vi "QcpTest.vi"() -> ()   [LabVIEW 2017]
uses:
  <userlib>/836-Library/System/QCP_V2/QCPSupportCode/QcpTests.ctl
  <userlib>/836-Library/System/QCP_V2/QCPSupportCode/QCP_GetDbl.vi
  <userlib>/836-Library/System/QCP_V2/QCPSupportCode/QCP_GetDblArr.vi
  <userlib>/836-Library/System/QCP_V2/QCPSupportCode/QCP_SetDbl.vi
panel:
  out "Numeric":i32
  out "All Tests Passed":bool
  out "Last Test Run":T1
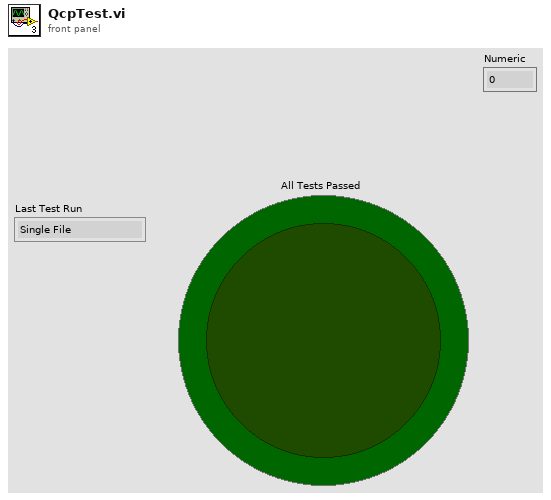
[diagram p1: front panel]
types:
  T1 = typedef "QcpTests.ctl" = enum16{"Single File", "Multiple FIle", "Tuning Mode", "Write FIle", "Same Name Prot On", "Same Name Prot Off", "NUM_TESTS"}
  T2 = typedef "QCP_RefNum.ctl" = cluster{"Data Value Refnum":refnum<data-value>, "semaphore":T3}
  T3 = typedef "Semaphore RefNum" = refnum<k1>
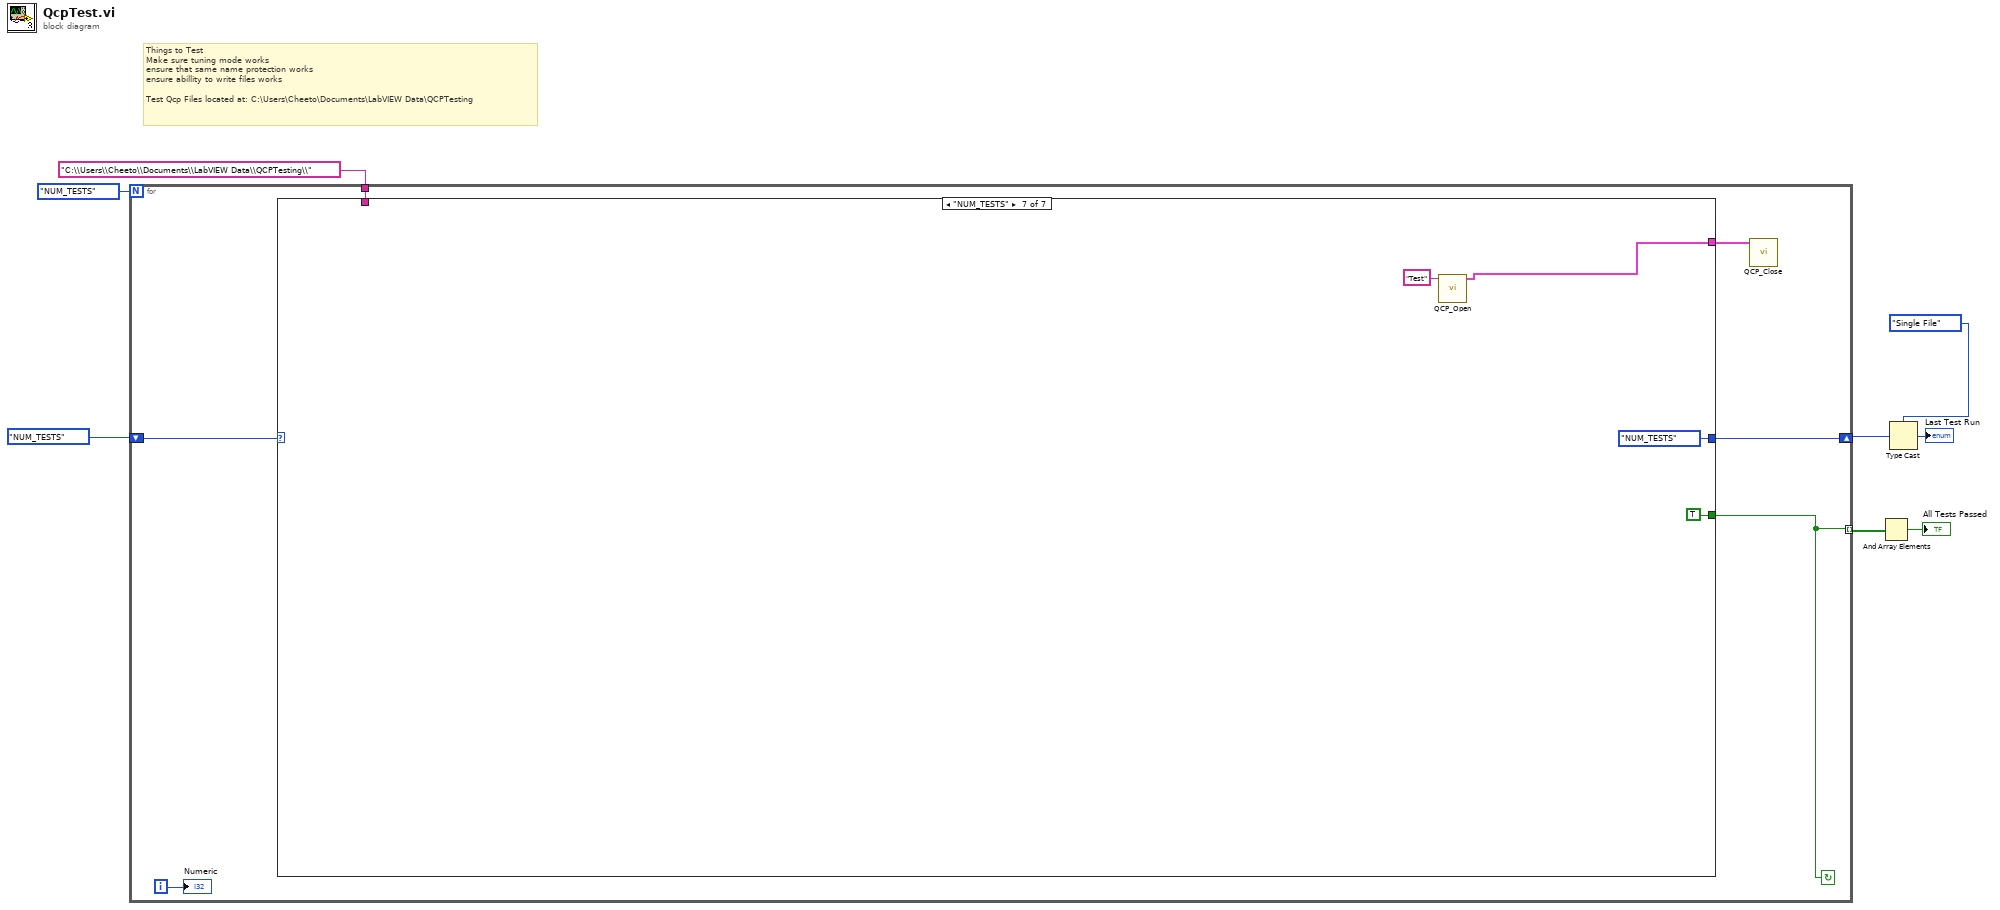
[diagram p0: block diagram]
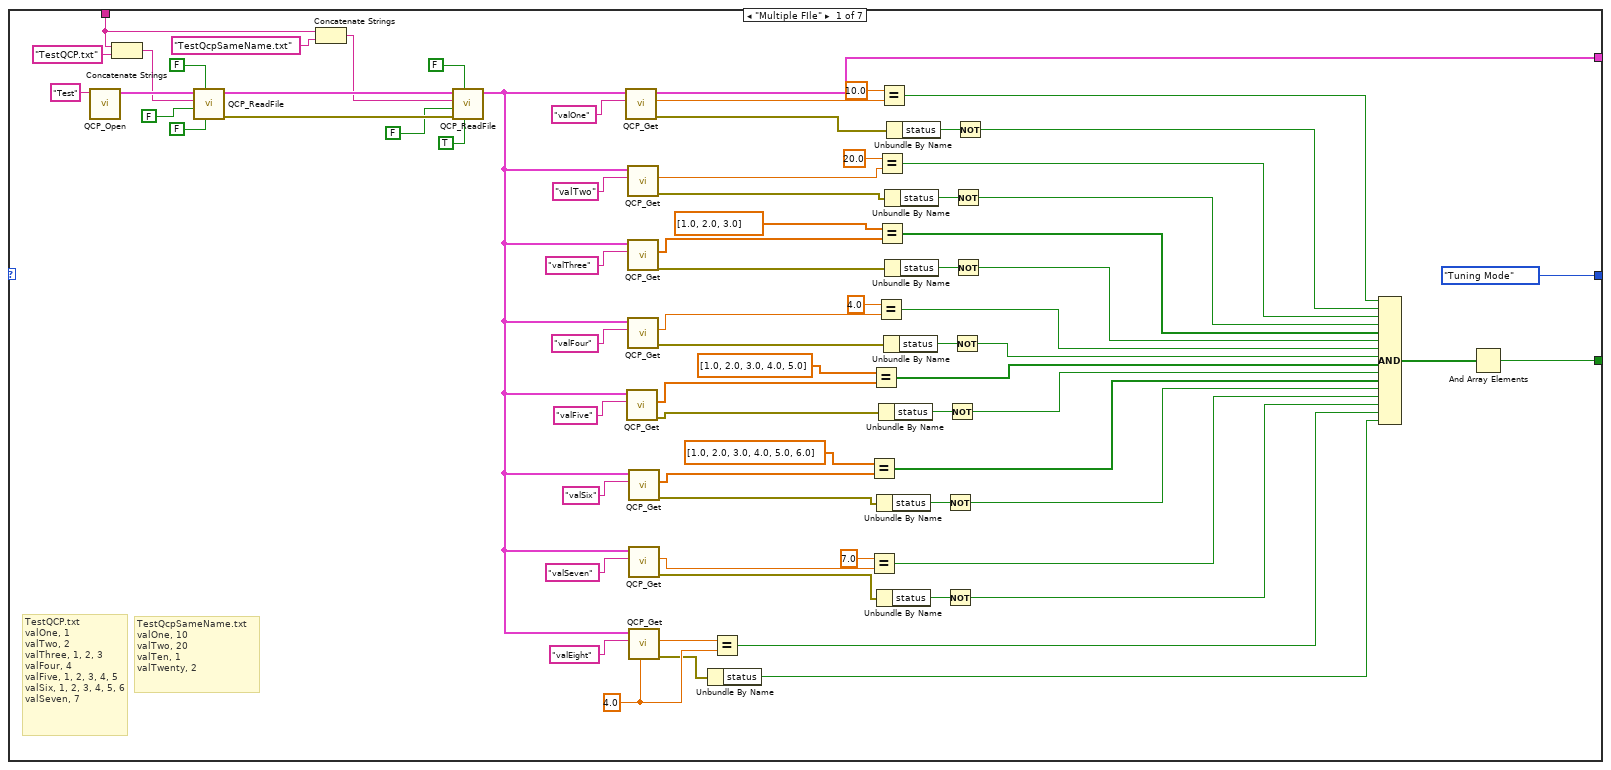
[diagram p2: hidden frame]
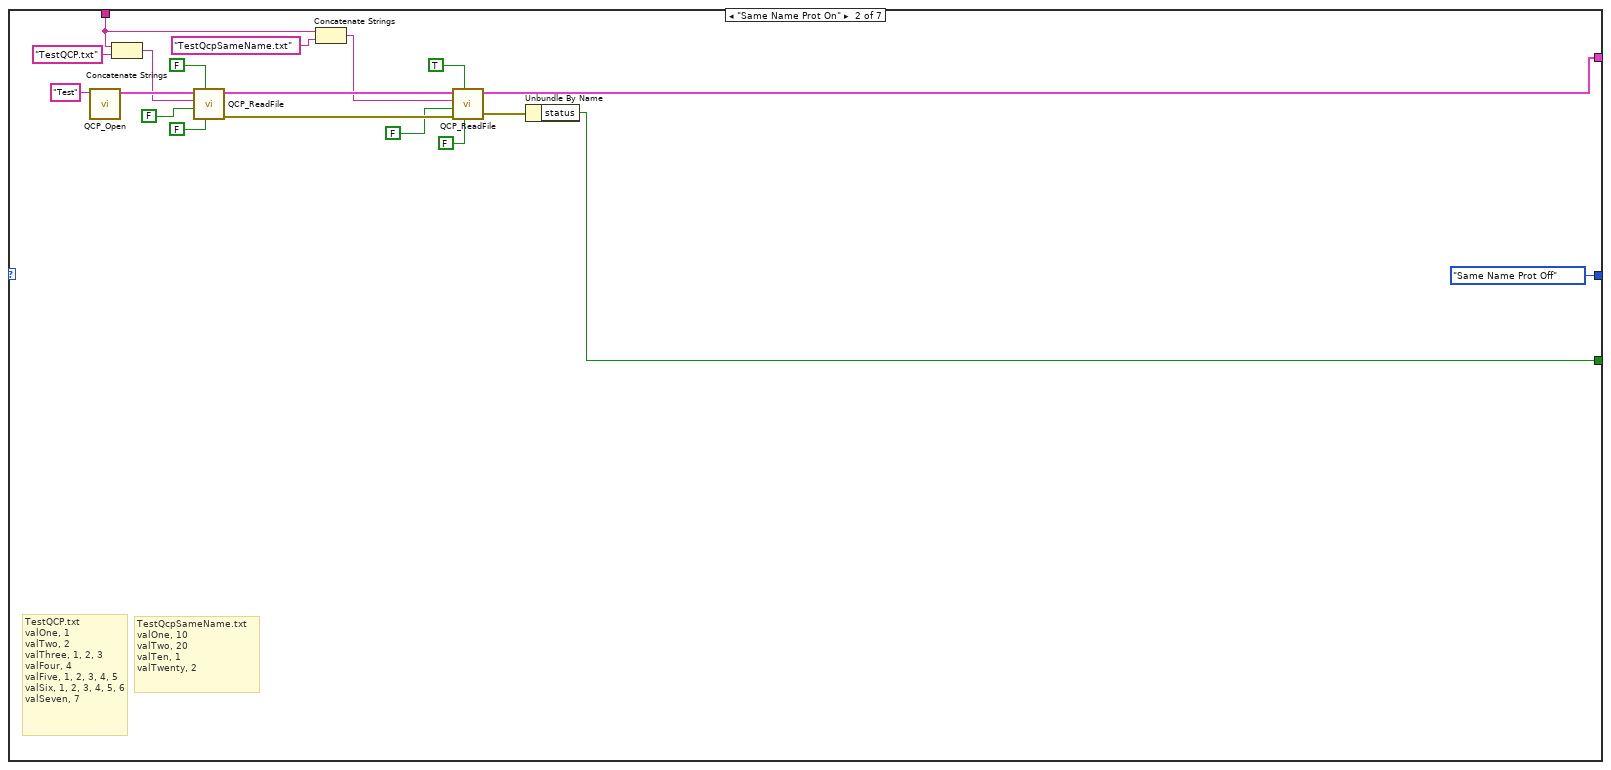
[diagram p3: hidden frame]
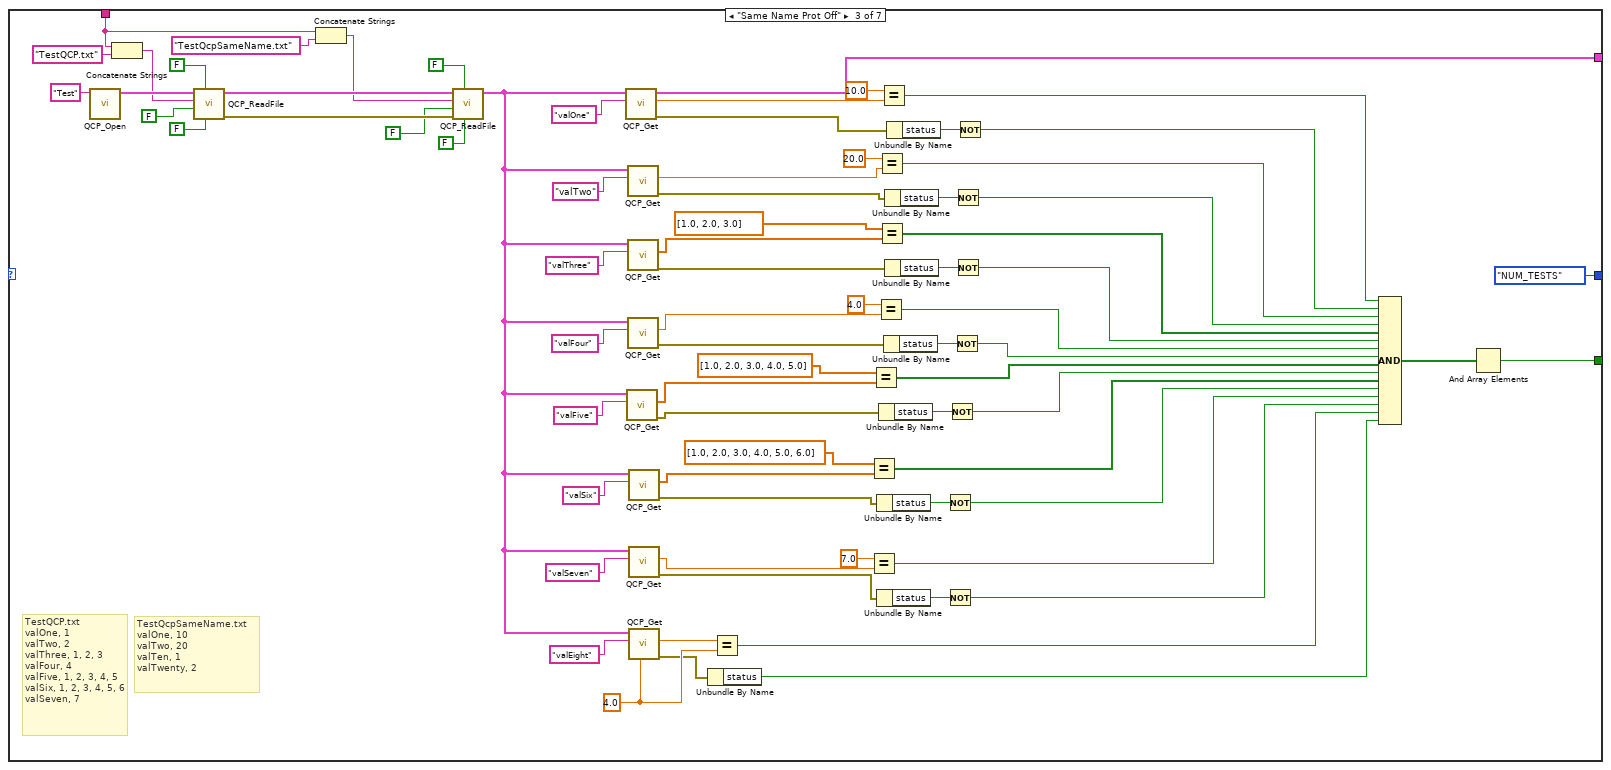
[diagram p4: hidden frame]
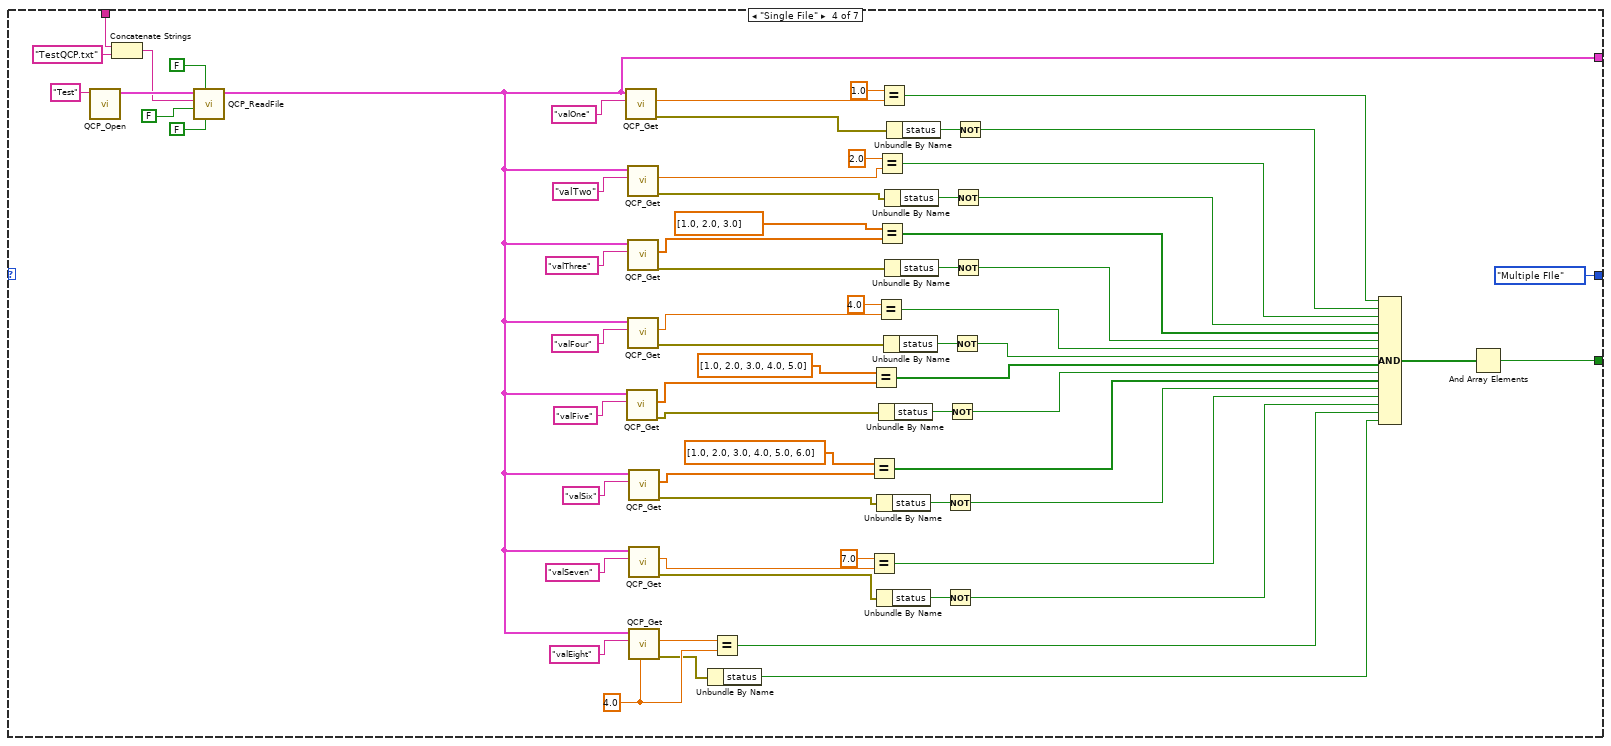
[diagram p5: hidden frame]
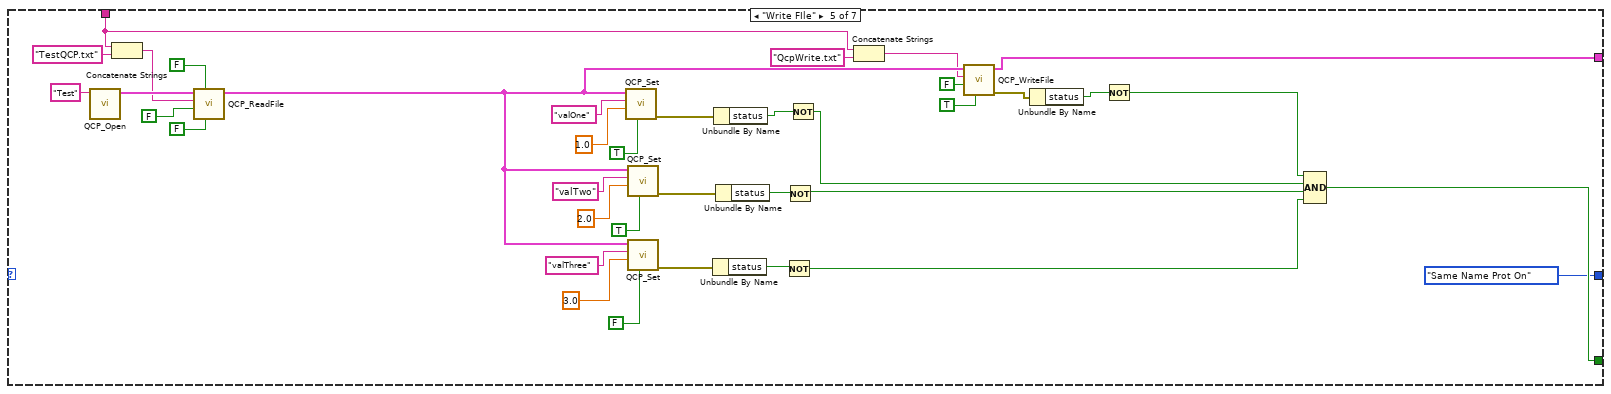
[diagram p6: hidden frame]
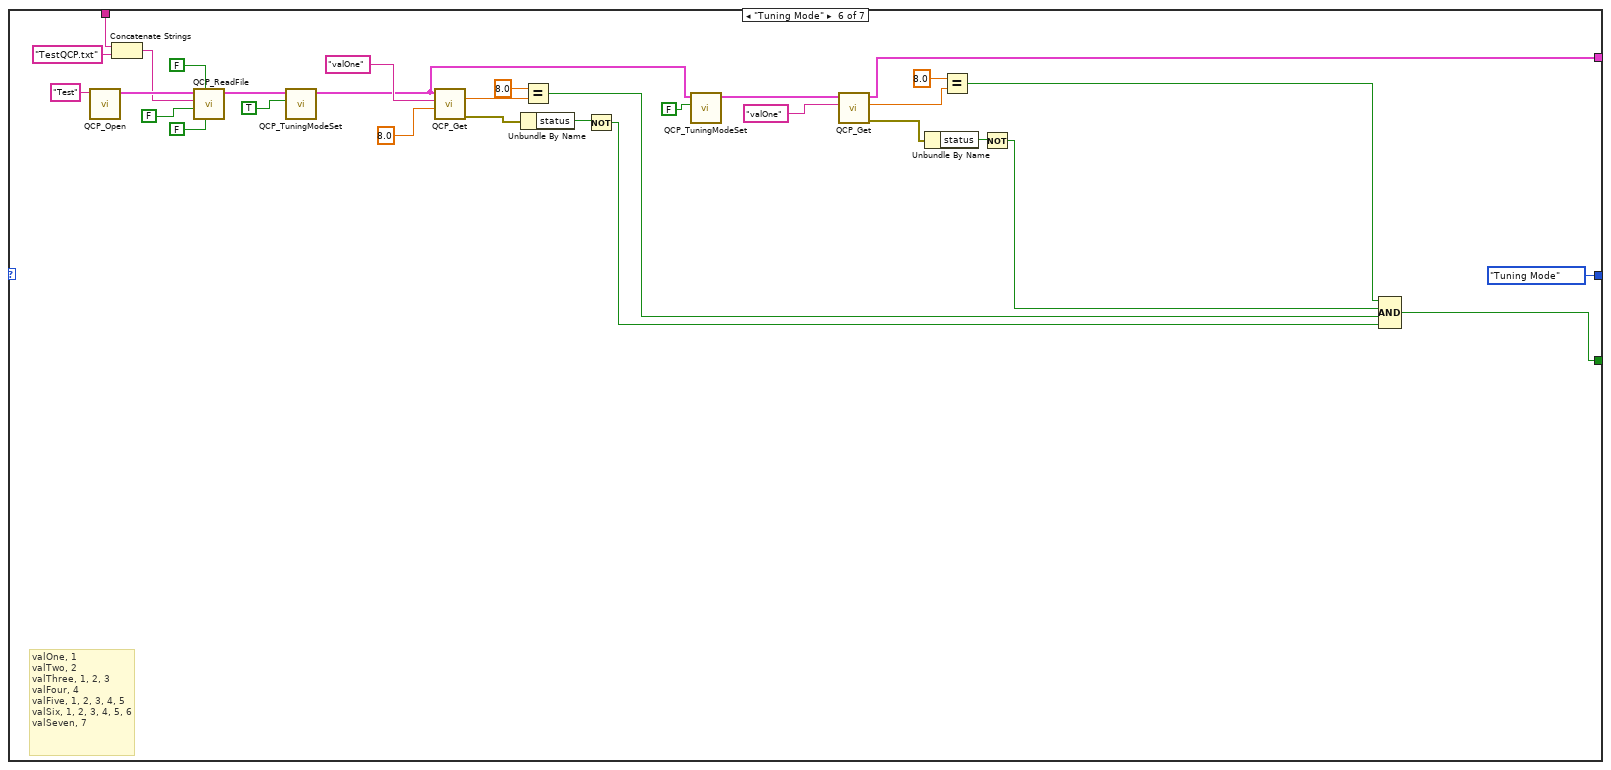
[diagram p7: hidden frame]
diagram:
  # "Things to Test\nMake sure tuning mode works\nensure that same name protection works\nensure abillity to write files works\n\nTest Qcp Files located at: C:\\Users\\Cheeto\\Documents\\LabVIEW Data\\QCPTesting"
  n1 = for {
    N: QcpTests."NUM_TESTS" -> [_]
    shift-right: [w10] -> w6
    shift-left: QcpTests."NUM_TESTS" -> [w11]
    tunnel: "C:\\Users\\Cheeto\\Documents\\LabVIEW Data\\QCPTesting\\" -> [w14]
    tunnel: [w12] -> w3 mode=indexing
    i -> [w9]
    stop <- w12 continue-if-true
    n2 = case shown="\"NUM_TESTS\"" w11 {
      tunnel: w14 -> [w19 w96 w113 w186 w267 w310 _]
      tunnel: [w26 w92 w120 w187 w252 w311 TRUE ("status")] -> w12
      tunnel: [w16 w91 w110 w185 w262 w296 w321] -> w13
      tunnel: [QcpTests."Tuning Mode" QcpTests."Same Name Prot Off" QcpTests."NUM_TESTS" QcpTests."Multiple FIle" QcpTests."Same Name Prot On" QcpTests."Tuning Mode" QcpTests."NUM_TESTS"] -> w10
      frame "Multiple FIle" {
        w73 = 4.0 ("Default Value")
        # "TestQcpSameName.txt\nvalOne, 10\nvalTwo, 20\nvalTen, 1\nvalTwenty, 2"
        # "TestQCP.txt\nvalOne, 1\nvalTwo, 2\nvalThree, 1, 2, 3\nvalFour, 4\nvalFive, 1, 2, 3, 4, 5\nvalSix, 1, 2, 3, 4, 5, 6\nvalSeven, 7"
        n3 = call <userlib>:"QCP_Open.vi"("Name"="Test") -> ("QCP_DevRef_Out"=w88:T2)  [unwired: 9 in, 1 out]
        n4 = Concatenate Strings(w19, "TestQCP.txt" ("string")) -> (w84:string)
        n5 = call <userlib>:"QCP_ReadFile.vi"("Overrite Existing Data?"=FALSE, "Same Name Fail?"=FALSE, "Path Relative?"=FALSE, "Path"=w84, "QCP_DevRef_In"=w88) -> ("error out"=w21:errorcluster, "QCP_DevRef_Out"=w24:T2)  [unwired: 5 in]
        n6 = Concatenate Strings(w19, "TestQcpSameName.txt" ("string")) -> (w17:string)
        n7 = call <userlib>:"QCP_ReadFile.vi"("Overrite Existing Data?"=TRUE, "Same Name Fail?"=FALSE, "error in"=w21, "Path Relative?"=FALSE, "Path"=w17, "QCP_DevRef_In"=w24) -> ("QCP_DevRef_Out"=w25:T2)  [unwired: 4 in, 1 out]
        n8 = call-poly <userlib>:"QCP_Get.vi"("Value Name"="valOne", "QCP_DevRef_In"=w25) -> ("error out"=w69:errorcluster, "Value"=w71:dbl, "QCP_DevRef_Out"=w16:T2)  [unwired: 7 in]
        n9 = call-poly <userlib>:"QCP_Get.vi"("Value Name"="valFive", "QCP_DevRef_In"=w25) -> ("error out"=w50:errorcluster, "Values"=w52:dbl[])  [unwired: 7 in, 1 out]
        n10 = call-poly <userlib>:"QCP_Get.vi"("Value Name"="valTwo", "QCP_DevRef_In"=w25) -> ("error out"=w59:errorcluster, "Value"=w61:dbl)  [unwired: 7 in, 1 out]
        n11 = call-poly <userlib>:"QCP_Get.vi"("Value Name"="valThree", "QCP_DevRef_In"=w25) -> ("error out"=w56:errorcluster, "Values"=w58:dbl[])  [unwired: 7 in, 1 out]
        n12 = call-poly <userlib>:"QCP_Get.vi"("Value Name"="valFour", "QCP_DevRef_In"=w25) -> ("error out"=w53:errorcluster, "Value"=w55:dbl)  [unwired: 7 in, 1 out]
        n13 = call-poly <userlib>:"QCP_Get.vi"("Value Name"="valSix", "QCP_DevRef_In"=w25) -> ("error out"=w48:errorcluster, "Values"=w49:dbl[])  [unwired: 7 in, 1 out]
        n14 = call-poly <userlib>:"QCP_Get.vi"("Value Name"="valSeven", "QCP_DevRef_In"=w25) -> ("error out"=w46:errorcluster, "Value"=w47:dbl)  [unwired: 7 in, 1 out]
        n15 = call-poly <userlib>:"QCP_Get.vi"("Default Value"=w73, "Value Name"="valEight", "QCP_DevRef_In"=w25) -> ("error out"=w72:errorcluster, "Value"=w74:dbl)  [unwired: 6 in, 1 out]
        n16 = Unbundle By Name(w72) -> ("status"=w28:bool)
        n17 = Equal?(x=w74, y=w73) -> (x = y?=w29:bool)
        n18 = Equal?(x=dbl[] [1.0, 2.0, 3.0, 4.0, 5.0, 6.0], y=w49) -> (x = y?=w33:bool[])
        n19 = Equal?(x=7.0, y=w47) -> (x = y?=w31:bool)
        n20 = Equal?(x=dbl[] [1.0, 2.0, 3.0, 4.0, 5.0], y=w52) -> (x = y?=w35:bool[])
        n21 = Equal?(x=4.0, y=w55) -> (x = y?=w37:bool)
        n22 = Equal?(x=20.0, y=w61) -> (x = y?=w41:bool)
        n23 = Equal?(x=dbl[] [1.0, 2.0, 3.0], y=w58) -> (x = y?=w39:bool[])
        n24 = Unbundle By Name(w48) -> ("status"=w63:bool)
        n25 = Unbundle By Name(w46) -> ("status"=w62:bool)
        n26 = Equal?(x=10.0, y=w71) -> (x = y?=w43:bool)
        n27 = Unbundle By Name(w50) -> ("status"=w64:bool)
        n28 = Unbundle By Name(w53) -> ("status"=w65:bool)
        n29 = Unbundle By Name(w59) -> ("status"=w67:bool)
        n30 = Unbundle By Name(w56) -> ("status"=w66:bool)
        n31 = Unbundle By Name(w69) -> ("status"=w68:bool)
        n32 = Not(x=w63) -> (.not. x?=w32:bool)
        n33 = Not(x=w62) -> (.not. x?=w30:bool)
        n34 = Not(x=w64) -> (.not. x?=w34:bool)
        n35 = Not(x=w65) -> (.not. x?=w36:bool)
        n36 = Not(x=w67) -> (.not. x?=w40:bool)
        n37 = Not(x=w66) -> (.not. x?=w38:bool)
        n38 = Not(x=w68) -> (.not. x?=w42:bool)
        n39 = Compound Arithmetic op=AND(w43, w42, w41, w40, w39, w38, w37, w36, w35, w34, w33, w32, w31, w30, w29, w28) -> (w27:bool[])
        n40 = And Array Elements(Boolean array=w27) -> (logical AND=w26:bool)
      }
      frame "Same Name Prot On" {
        # "TestQcpSameName.txt\nvalOne, 10\nvalTwo, 20\nvalTen, 1\nvalTwenty, 2"
        # "TestQCP.txt\nvalOne, 1\nvalTwo, 2\nvalThree, 1, 2, 3\nvalFour, 4\nvalFive, 1, 2, 3, 4, 5\nvalSix, 1, 2, 3, 4, 5, 6\nvalSeven, 7"
        n41 = call <userlib>:"QCP_Open.vi"("Name"="Test") -> ("QCP_DevRef_Out"=w107:T2)  [unwired: 9 in, 1 out]
        n42 = Concatenate Strings(w96, "TestQCP.txt" ("string")) -> (w103:string)
        n43 = call <userlib>:"QCP_ReadFile.vi"("Overrite Existing Data?"=FALSE, "Same Name Fail?"=FALSE, "Path Relative?"=FALSE, "Path"=w103, "QCP_DevRef_In"=w107) -> ("error out"=w98:errorcluster, "QCP_DevRef_Out"=w101:T2)  [unwired: 5 in]
        n44 = Concatenate Strings(w96, "TestQcpSameName.txt" ("string")) -> (w94:string)
        n45 = call <userlib>:"QCP_ReadFile.vi"("Overrite Existing Data?"=FALSE, "Same Name Fail?"=TRUE, "error in"=w98, "Path Relative?"=FALSE, "Path"=w94, "QCP_DevRef_In"=w101) -> ("error out"=w93:errorcluster, "QCP_DevRef_Out"=w91:T2)  [unwired: 4 in]
        n46 = Unbundle By Name(w93) -> ("status"=w92:bool)
      }
      frame "Same Name Prot Off" {
        w167 = 4.0 ("Default Value")
        # "TestQcpSameName.txt\nvalOne, 10\nvalTwo, 20\nvalTen, 1\nvalTwenty, 2"
        # "TestQCP.txt\nvalOne, 1\nvalTwo, 2\nvalThree, 1, 2, 3\nvalFour, 4\nvalFive, 1, 2, 3, 4, 5\nvalSix, 1, 2, 3, 4, 5, 6\nvalSeven, 7"
        n47 = call <userlib>:"QCP_Open.vi"("Name"="Test") -> ("QCP_DevRef_Out"=w182:T2)  [unwired: 9 in, 1 out]
        n48 = Concatenate Strings(w113, "TestQCP.txt" ("string")) -> (w178:string)
        n49 = call <userlib>:"QCP_ReadFile.vi"("Overrite Existing Data?"=FALSE, "Same Name Fail?"=FALSE, "Path Relative?"=FALSE, "Path"=w178, "QCP_DevRef_In"=w182) -> ("error out"=w115:errorcluster, "QCP_DevRef_Out"=w118:T2)  [unwired: 5 in]
        n50 = Concatenate Strings(w113, "TestQcpSameName.txt" ("string")) -> (w111:string)
        n51 = call <userlib>:"QCP_ReadFile.vi"("Overrite Existing Data?"=FALSE, "Same Name Fail?"=FALSE, "error in"=w115, "Path Relative?"=FALSE, "Path"=w111, "QCP_DevRef_In"=w118) -> ("QCP_DevRef_Out"=w119:T2)  [unwired: 4 in, 1 out]
        n52 = call-poly <userlib>:"QCP_Get.vi"("Value Name"="valOne", "QCP_DevRef_In"=w119) -> ("error out"=w163:errorcluster, "Value"=w165:dbl, "QCP_DevRef_Out"=w110:T2)  [unwired: 7 in]
        n53 = call-poly <userlib>:"QCP_Get.vi"("Value Name"="valFive", "QCP_DevRef_In"=w119) -> ("error out"=w144:errorcluster, "Values"=w146:dbl[])  [unwired: 7 in, 1 out]
        n54 = call-poly <userlib>:"QCP_Get.vi"("Value Name"="valTwo", "QCP_DevRef_In"=w119) -> ("error out"=w153:errorcluster, "Value"=w155:dbl)  [unwired: 7 in, 1 out]
        n55 = call-poly <userlib>:"QCP_Get.vi"("Value Name"="valThree", "QCP_DevRef_In"=w119) -> ("error out"=w150:errorcluster, "Values"=w152:dbl[])  [unwired: 7 in, 1 out]
        n56 = call-poly <userlib>:"QCP_Get.vi"("Value Name"="valFour", "QCP_DevRef_In"=w119) -> ("error out"=w147:errorcluster, "Value"=w149:dbl)  [unwired: 7 in, 1 out]
        n57 = call-poly <userlib>:"QCP_Get.vi"("Value Name"="valSix", "QCP_DevRef_In"=w119) -> ("error out"=w142:errorcluster, "Values"=w143:dbl[])  [unwired: 7 in, 1 out]
        n58 = call-poly <userlib>:"QCP_Get.vi"("Value Name"="valSeven", "QCP_DevRef_In"=w119) -> ("error out"=w140:errorcluster, "Value"=w141:dbl)  [unwired: 7 in, 1 out]
        n59 = call-poly <userlib>:"QCP_Get.vi"("Default Value"=w167, "Value Name"="valEight", "QCP_DevRef_In"=w119) -> ("error out"=w166:errorcluster, "Value"=w168:dbl)  [unwired: 6 in, 1 out]
        n60 = Unbundle By Name(w166) -> ("status"=w122:bool)
        n61 = Equal?(x=w168, y=w167) -> (x = y?=w123:bool)
        n62 = Equal?(x=dbl[] [1.0, 2.0, 3.0, 4.0, 5.0, 6.0], y=w143) -> (x = y?=w127:bool[])
        n63 = Equal?(x=7.0, y=w141) -> (x = y?=w125:bool)
        n64 = Equal?(x=dbl[] [1.0, 2.0, 3.0, 4.0, 5.0], y=w146) -> (x = y?=w129:bool[])
        n65 = Equal?(x=4.0, y=w149) -> (x = y?=w131:bool)
        n66 = Equal?(x=20.0, y=w155) -> (x = y?=w135:bool)
        n67 = Equal?(x=dbl[] [1.0, 2.0, 3.0], y=w152) -> (x = y?=w133:bool[])
        n68 = Unbundle By Name(w142) -> ("status"=w157:bool)
        n69 = Unbundle By Name(w140) -> ("status"=w156:bool)
        n70 = Equal?(x=10.0, y=w165) -> (x = y?=w137:bool)
        n71 = Unbundle By Name(w144) -> ("status"=w158:bool)
        n72 = Unbundle By Name(w147) -> ("status"=w159:bool)
        n73 = Unbundle By Name(w153) -> ("status"=w161:bool)
        n74 = Unbundle By Name(w150) -> ("status"=w160:bool)
        n75 = Unbundle By Name(w163) -> ("status"=w162:bool)
        n76 = Not(x=w157) -> (.not. x?=w126:bool)
        n77 = Not(x=w156) -> (.not. x?=w124:bool)
        n78 = Not(x=w158) -> (.not. x?=w128:bool)
        n79 = Not(x=w159) -> (.not. x?=w130:bool)
        n80 = Not(x=w161) -> (.not. x?=w134:bool)
        n81 = Not(x=w160) -> (.not. x?=w132:bool)
        n82 = Not(x=w162) -> (.not. x?=w136:bool)
        n83 = Compound Arithmetic op=AND(w137, w136, w135, w134, w133, w132, w131, w130, w129, w128, w127, w126, w125, w124, w123, w122) -> (w121:bool[])
        n84 = And Array Elements(Boolean array=w121) -> (logical AND=w120:bool)
      }
      frame "Single File" {
        w234 = 4.0 ("Default Value")
        n85 = call <userlib>:"QCP_Open.vi"("Name"="Test") -> ("QCP_DevRef_Out"=w249:T2)  [unwired: 9 in, 1 out]
        n86 = Concatenate Strings(w186, "TestQCP.txt" ("string")) -> (w245:string)
        n87 = call <userlib>:"QCP_ReadFile.vi"("Overrite Existing Data?"=FALSE, "Same Name Fail?"=FALSE, "Path Relative?"=FALSE, "Path"=w245, "QCP_DevRef_In"=w249) -> ("QCP_DevRef_Out"=w185:T2)  [unwired: 5 in, 1 out]
        n88 = call-poly <userlib>:"QCP_Get.vi"("Value Name"="valOne", "QCP_DevRef_In"=w185) -> ("error out"=w230:errorcluster, "Value"=w232:dbl)  [unwired: 7 in, 1 out]
        n89 = call-poly <userlib>:"QCP_Get.vi"("Value Name"="valFive", "QCP_DevRef_In"=w185) -> ("error out"=w211:errorcluster, "Values"=w213:dbl[])  [unwired: 7 in, 1 out]
        n90 = call-poly <userlib>:"QCP_Get.vi"("Value Name"="valTwo", "QCP_DevRef_In"=w185) -> ("error out"=w220:errorcluster, "Value"=w222:dbl)  [unwired: 7 in, 1 out]
        n91 = call-poly <userlib>:"QCP_Get.vi"("Value Name"="valThree", "QCP_DevRef_In"=w185) -> ("error out"=w217:errorcluster, "Values"=w219:dbl[])  [unwired: 7 in, 1 out]
        n92 = call-poly <userlib>:"QCP_Get.vi"("Value Name"="valFour", "QCP_DevRef_In"=w185) -> ("error out"=w214:errorcluster, "Value"=w216:dbl)  [unwired: 7 in, 1 out]
        n93 = call-poly <userlib>:"QCP_Get.vi"("Value Name"="valSix", "QCP_DevRef_In"=w185) -> ("error out"=w209:errorcluster, "Values"=w210:dbl[])  [unwired: 7 in, 1 out]
        n94 = call-poly <userlib>:"QCP_Get.vi"("Value Name"="valSeven", "QCP_DevRef_In"=w185) -> ("error out"=w207:errorcluster, "Value"=w208:dbl)  [unwired: 7 in, 1 out]
        n95 = call-poly <userlib>:"QCP_Get.vi"("Default Value"=w234, "Value Name"="valEight", "QCP_DevRef_In"=w185) -> ("error out"=w233:errorcluster, "Value"=w235:dbl)  [unwired: 6 in, 1 out]
        n96 = Unbundle By Name(w233) -> ("status"=w189:bool)
        n97 = Equal?(x=w235, y=w234) -> (x = y?=w190:bool)
        n98 = Equal?(x=dbl[] [1.0, 2.0, 3.0, 4.0, 5.0, 6.0], y=w210) -> (x = y?=w194:bool[])
        n99 = Equal?(x=7.0, y=w208) -> (x = y?=w192:bool)
        n100 = Equal?(x=dbl[] [1.0, 2.0, 3.0, 4.0, 5.0], y=w213) -> (x = y?=w196:bool[])
        n101 = Equal?(x=4.0, y=w216) -> (x = y?=w198:bool)
        n102 = Equal?(x=2.0, y=w222) -> (x = y?=w202:bool)
        n103 = Equal?(x=dbl[] [1.0, 2.0, 3.0], y=w219) -> (x = y?=w200:bool[])
        n104 = Unbundle By Name(w209) -> ("status"=w224:bool)
        n105 = Unbundle By Name(w207) -> ("status"=w223:bool)
        n106 = Equal?(x=1.0, y=w232) -> (x = y?=w204:bool)
        n107 = Unbundle By Name(w211) -> ("status"=w225:bool)
        n108 = Unbundle By Name(w214) -> ("status"=w226:bool)
        n109 = Unbundle By Name(w220) -> ("status"=w228:bool)
        n110 = Unbundle By Name(w217) -> ("status"=w227:bool)
        n111 = Unbundle By Name(w230) -> ("status"=w229:bool)
        n112 = Not(x=w224) -> (.not. x?=w193:bool)
        n113 = Not(x=w223) -> (.not. x?=w191:bool)
        n114 = Not(x=w225) -> (.not. x?=w195:bool)
        n115 = Not(x=w226) -> (.not. x?=w197:bool)
        n116 = Not(x=w228) -> (.not. x?=w201:bool)
        n117 = Not(x=w227) -> (.not. x?=w199:bool)
        n118 = Not(x=w229) -> (.not. x?=w203:bool)
        n119 = Compound Arithmetic op=AND(w204, w203, w202, w201, w200, w199, w198, w197, w196, w195, w194, w193, w192, w191, w190, w189) -> (w188:bool[])
        n120 = And Array Elements(Boolean array=w188) -> (logical AND=w187:bool)
      }
      frame "Write FIle" {
        n121 = call <userlib>:"QCP_Open.vi"("Name"="Test") -> ("QCP_DevRef_Out"=w286:T2)  [unwired: 9 in, 1 out]
        n122 = Concatenate Strings(w267, "TestQCP.txt" ("string")) -> (w282:string)
        n123 = call <userlib>:"QCP_ReadFile.vi"("Overrite Existing Data?"=FALSE, "Same Name Fail?"=FALSE, "Path Relative?"=FALSE, "Path"=w282, "QCP_DevRef_In"=w286) -> ("QCP_DevRef_Out"=w268:T2)  [unwired: 5 in, 1 out]
        n124 = call-poly <userlib>:"QCP_Set.vi"("Add if New?"=TRUE, "Value"=1.0, "Name"="valOne" ("Value Name"), "QCP_DevRef_In"=w268) -> ("error out"=w272:errorcluster)  [unwired: 6 in, 1 out]
        n125 = call-poly <userlib>:"QCP_Set.vi"("Add if New?"=TRUE, "Value"=2.0, "Name"="valTwo" ("Value Name"), "QCP_DevRef_In"=w268) -> ("error out"=w273:errorcluster)  [unwired: 6 in, 1 out]
        n126 = call-poly <userlib>:"QCP_Set.vi"("Add if New?"=FALSE, "Value"=3.0, "Name"="valThree" ("Value Name"), "QCP_DevRef_In"=w268) -> ("error out"=w274:errorcluster)  [unwired: 6 in, 1 out]
        n127 = Unbundle By Name(w274) -> ("status"=w270:bool)
        n128 = Unbundle By Name(w272) -> ("status"=w271:bool)
        n129 = Unbundle By Name(w273) -> ("status"=w269:bool)
        n130 = Not(x=w270) -> (.not. x?=w253:bool)
        n131 = Not(x=w269) -> (.not. x?=w254:bool)
        n132 = Not(x=w271) -> (.not. x?=w255:bool)
        n133 = Concatenate Strings(w267, "QcpWrite.txt" ("string")) -> (w265:string)
        n134 = call <userlib>:"QCP_WriteFile.vi"("Overrite?"=TRUE, "Path relative?"=FALSE, "Path"=w265, "QCP_DevRef_In"=w268) -> ("error out"=w260:errorcluster, "QCP_DevRef_Out"=w262:T2)  [unwired: 6 in]
        n135 = Unbundle By Name(w260) -> ("status"=w261:bool)
        n136 = Not(x=w261) -> (.not. x?=w256:bool)
        n137 = Compound Arithmetic op=AND(w256, w255, w254, w253) -> (w252:bool)
      }
      frame "Tuning Mode" {
        # "valOne, 1\nvalTwo, 2\nvalThree, 1, 2, 3\nvalFour, 4\nvalFive, 1, 2, 3, 4, 5\nvalSix, 1, 2, 3, 4, 5, 6\nvalSeven, 7"
        n138 = call <userlib>:"QCP_Open.vi"("Name"="Test") -> ("QCP_DevRef_Out"=w317:T2)  [unwired: 9 in, 1 out]
        n139 = Concatenate Strings(w310, "TestQCP.txt" ("string")) -> (w313:string)
        n140 = call <userlib>:"QCP_ReadFile.vi"("Overrite Existing Data?"=FALSE, "Same Name Fail?"=FALSE, "Path Relative?"=FALSE, "Path"=w313, "QCP_DevRef_In"=w317) -> ("QCP_DevRef_Out"=w309:T2)  [unwired: 5 in, 1 out]
        n141 = call <userlib>:"QCP_TuningModeSet.vi"("On?"=TRUE, "QCP_DevRef_In"=w309) -> ("QCP_DevRef_Out"=w302:T2)  [unwired: 8 in, 1 out]
        n142 = call-poly <userlib>:"QCP_Get.vi"("Tuning Value"=8.0, "Value Name"="valOne", "QCP_DevRef_In"=w302) -> ("error out"=w303:errorcluster, "Value"=w305:dbl)  [unwired: 6 in, 1 out]
        n143 = Unbundle By Name(w303) -> ("status"=w293:bool)
        n144 = Equal?(x=8.0, y=w305) -> (x = y?=w290:bool)
        n145 = Not(x=w293) -> (.not. x?=w289:bool)
        n146 = call <userlib>:"QCP_TuningModeSet.vi"("On?"=FALSE, "QCP_DevRef_In"=w302) -> ("QCP_DevRef_Out"=w300:T2)  [unwired: 8 in, 1 out]
        n147 = call-poly <userlib>:"QCP_Get.vi"("Value Name"="valOne", "QCP_DevRef_In"=w300) -> ("error out"=w295:errorcluster, "Value"=w297:dbl, "QCP_DevRef_Out"=w296:T2)  [unwired: 7 in]
        n148 = Unbundle By Name(w295) -> ("status"=w294:bool)
        n149 = Equal?(x=8.0, y=w297) -> (x = y?=w292:bool)
        n150 = Not(x=w294) -> (.not. x?=w291:bool)
        n151 = Compound Arithmetic op=AND(w292, w291, w290, w289) -> (w311:bool)
      }
      frame "NUM_TESTS" {
        n152 = call <userlib>:"QCP_Open.vi"("Name"="Test") -> ("QCP_DevRef_Out"=w321:T2)  [unwired: 9 in, 1 out]
      }
    }
    n153 = call <userlib>:"QCP_Close.vi"("QCP_DevRef_In"=w13) -> ()  [unwired: 10 in, 1 out]
    "Numeric" <- w9
  }
  n154 = And Array Elements(Boolean array=w3) -> (logical AND=→"All Tests Passed":bool)
  n155 = Type Cast(type=QcpTests."Single File", x=w6) -> (*(type *) &x=→"Last Test Run":T1)
